vi "To Sample Line.vi"(8 "error in (no error)":errorcluster, 10 "Metric Name":string, 11 "Sample in":refnum<class "Sample.lvclass">) -> (0 "error out":errorcluster, 3 "Sample line":string)   [LabVIEW 2020, in "Metrics.lvlib" / "Sample.lvclass"]
uses:
  Sample.lvclass
  Sample.lvclass/Sample.ctl
  Read Value.vi
  Read Labels.vi
  Read Timestamp.vi
  utils/LV timestamp to unix.vi
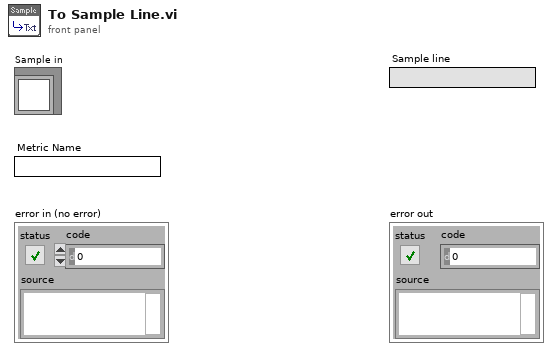
[diagram p1: front panel]
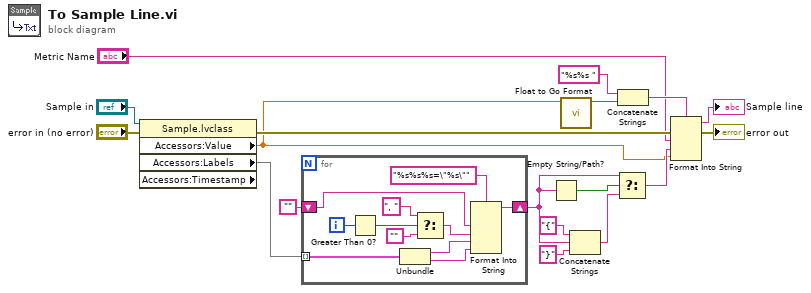
[diagram p0: block diagram]
diagram:
  n1 = property class="Sample.lvclass" props=["Accessors:Value", "Accessors:Labels", "Accessors:Timestamp"](reference="Sample in", error in="error in (no error)") -> (error out=w16:errorcluster, "Accessors:Value"=w4:dbl, "Accessors:Labels"=w2:map{string, string})  [unwired: 2 out]
  n2 = for {
    tunnel: w2 -> [w29] mode=indexing
    shift-right: [w20] -> w5
    shift-left: "" -> [w23]
    i -> [w27]
    n3 = Greater Than 0?(x=w27) -> (x > 0?=w26:bool)
    n4 = Unbundle(w29) -> ("labelname"=w21:string, "labelvalue"=w19:string)
    n5 = Select(t=", ", s=w26, f="") -> (s? t:f=w22:string)
    n6 = Format Into String(format string="%s%s%s=\"%s\"", w23, w22, w21, w19) -> (resulting string=w20:string)  [unwired: 2 in, 1 out]
  }
  n7 = Empty String/Path?(string/path=w5) -> (empty?=w17:bool)
  n8 = call "Float to Go Format.vi"("Float Value"=w4) -> ("Go Format"=w3:string)  [unwired: 10 in]
  n9 = Concatenate Strings("{" ("string"), w5, "}" ("string")) -> (w7:string)
  n10 = Select(t=w5, s=w17, f=w7) -> (s? t:f=w18:string)
  n11 = Concatenate Strings("%s%s " ("string"), w3) -> (w11:string)
  n12 = Format Into String(format string=w11, error in=w16, "Metric Name", w18, w4) -> (resulting string=→"Sample line":string, error out=→"error out":errorcluster)  [unwired: 1 in]
